vi "Write Configuration dict.vi"(8 "error in (no error)":errorcluster, 9 "Config Name":string, 10 "Config.lvclass":refnum<class "Config.lvclass">, 11 "Control in":refnum<class "Control-Server.lvclass">) -> (0 "error out":errorcluster, 3 "Control out":refnum<class "Control-Server.lvclass">)   [LabVIEW 2015, in "Control-Server.lvclass"]
uses:
  Control-Server.lvclass
  Config/Config.lvclass
  Control-Server.lvclass/Control-Server.ctl
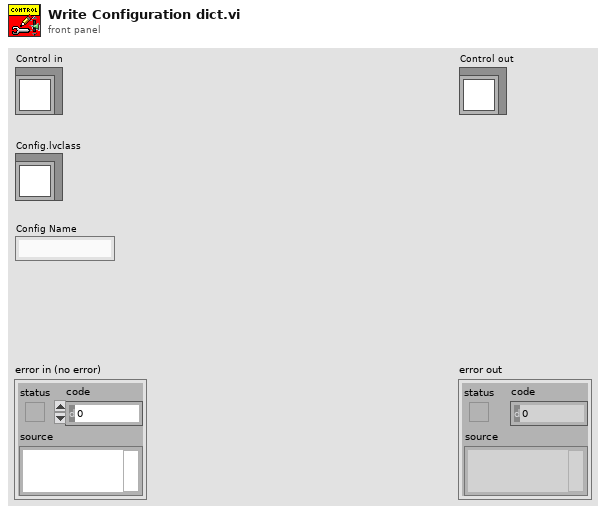
[diagram p1: front panel]
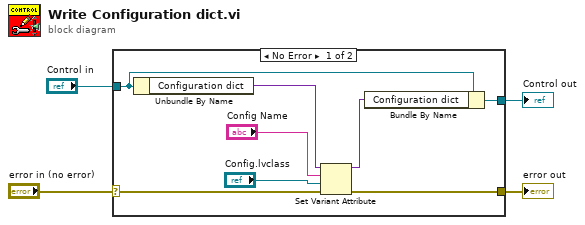
[diagram p0: block diagram]
diagram:
  n1 = case shown="No Error" "error in (no error)" {
    selector: "error in (no error)" -> [w9 w13]
    tunnel: [w8 w13] -> w3
    tunnel: [w12 w14] -> w1
    tunnel: "Control in" -> [w11 w14]
    frame No Error {
      n2 = Unbundle By Name(w11) -> ("Configuration dict"=w10:variant)
      n3 = Set Variant Attribute(Variant=w10, name="Config Name", value="Config.lvclass", error in=w9) -> (Variant out=w5:variant, error out=w8:errorcluster)  [unwired: 1 out]
      n4 = Bundle By Name(cluster=w11, "Configuration dict"=w5) -> (w12:refnum<class "Control-Server.lvclass">)
    }
    frame Error {
    }
  }
  "error out" <- w3
  "Control out" <- w1
